vi "Gaussian White Noise.vi"(7 "initialize?":bool=TRUE, 9 "seed":i32=-1, 10 "standard deviation":dbl=1.0000000000000002 format="%0.2f", 11 "samples":i32=128) -> (0 "error":i32, 3 "Gaussian noise pattern":dbl[](array[numeric]))   [LabVIEW 2020, in "NI_AALBase.lvlib"]
doc: "Generates a Gaussian-distributed, pseudorandom pattern whose statistical profile is (mu, sigma) = (0, s), where s is <B>standard deviation</B>."
uses:
  NI_AALBase.lvlib
  <resource>/lvanlys.dll
panel:
  # "Gaussian White Noise"
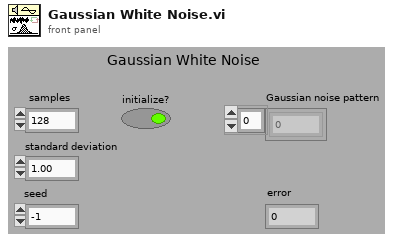
[diagram p1: front panel]
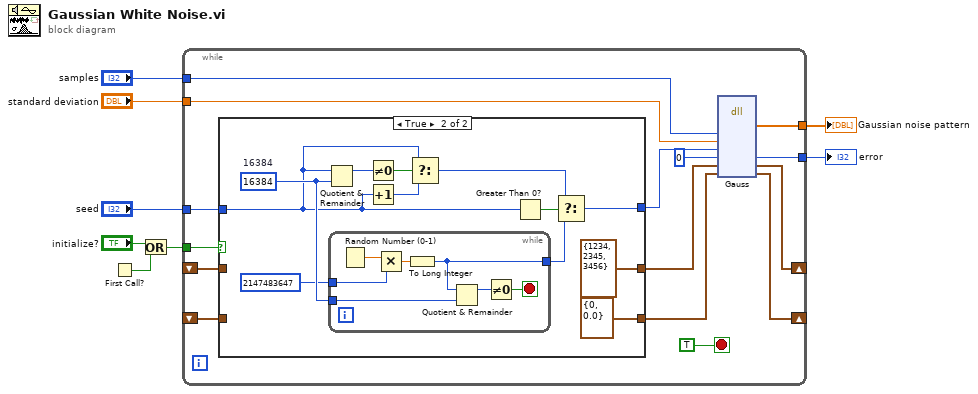
[diagram p0: block diagram]
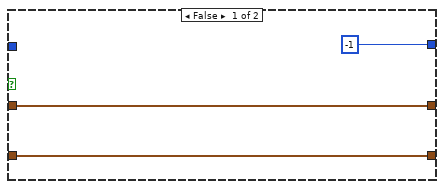
[diagram p2: hidden frame]
diagram:
  n1 = First Call?() -> (First Call?: T/F=w2:bool)
  n2 = Or(x="initialize?", y=w2) -> (x .or. y?=w1:bool)
  n3 = while {
    shift-right: [w14] -> _
    shift-left: _ -> [w17]
    tunnel: w1 -> [w11]
    shift-right: [w12] -> _
    shift-left: _ -> [w16]
    tunnel: "seed" -> [w19]
    tunnel: "standard deviation" -> [w21]
    tunnel: "samples" -> [w20]
    tunnel: [w10] -> w5
    tunnel: [w9] -> w4
    stop <- TRUE stop-if-true
    n4 = case shown="True" w11 {
      tunnel: [w26 cluster{"xSeed":i32, "ySeed":i32, "zSeed":i32} {"xSeed"=1234, "ySeed"=2345, "zSeed"=3456} ("RNGState")] -> w15
      tunnel: [-1 ("seed") w28] -> w18
      tunnel: w19 -> [_ w27]
      tunnel: [w25 cluster{i32, dbl} {0, 0.0}] -> w13
      tunnel: w17 -> [w26 _]
      tunnel: w16 -> [w25 _]
      frame False {
      }
      frame True {
        w30 = 16384  # 16384
        n5 = Quotient & Remainder(x=w27, y=w30) -> (x-y*floor(x/y)=w35:i32)  [unwired: 1 out]
        n6 = while {
          tunnel: [w43] -> w31
          tunnel: w30 -> [w42]
          tunnel: 2147483647 ("x") -> [w39]
          stop <- w40 stop-if-true
          n7 = Random Number (0-1)() -> (number: 0 to 1=w44:dbl)
          n8 = Multiply(x=w44, y=w39) -> (x*y=w45:dbl)
          n9 = To Long Integer(number=w45) -> (32bit integer=w43:i32)
          n10 = Quotient & Remainder(x=w43, y=w42) -> (x-y*floor(x/y)=w41:i32)  [unwired: 1 out]
          n11 = Not Equal To 0?(x=w41) -> (x != 0?=w40:bool)
        }
        n12 = Not Equal To 0?(x=w35) -> (x != 0?=w34:bool)
        n13 = Increment(x=w27) -> (x+1=w33:i32)
        n14 = Select(t=w27, s=w34, f=w33) -> (s? t:f=w32:i32)
        n15 = Greater Than 0?(x=w27) -> (x > 0?=w36:bool)
        n16 = Select(t=w32, s=w36, f=w31) -> (s? t:f=w28:i32)
      }
    }
    n17 = dll-call lib="C:/Program Files (x86)/National Instruments/LabVIEW 2020/resource/lvanlys.*" fn="Gauss"("size"=w20, "stanDev"=w21, "theSeed"=w18, "dsperr"=0, "rngState"=w15, "gaussState"=w13) -> ("xH"=w9:dbl[], "dsperr"=w10:i32, "rngState"=w14:cluster{"xSeed":i32, "ySeed":i32, "zSeed":i32}, "gaussState"=w12:cluster{i32, dbl})  [unwired: 6 in, 4 out]
  }
  "error" <- w5
  "Gaussian noise pattern" <- w4
